vi "uA_build_version.vi"(8 "error in (no error)":errorcluster, 10 "name or relative path":string="Power_Measurement_kit_V2.exe", 11 "path":path) -> (0 "error out":errorcluster, 2 "status":bool, 3 "FileVersion":string)   [LabVIEW 2015]
panel:
  out "string":string
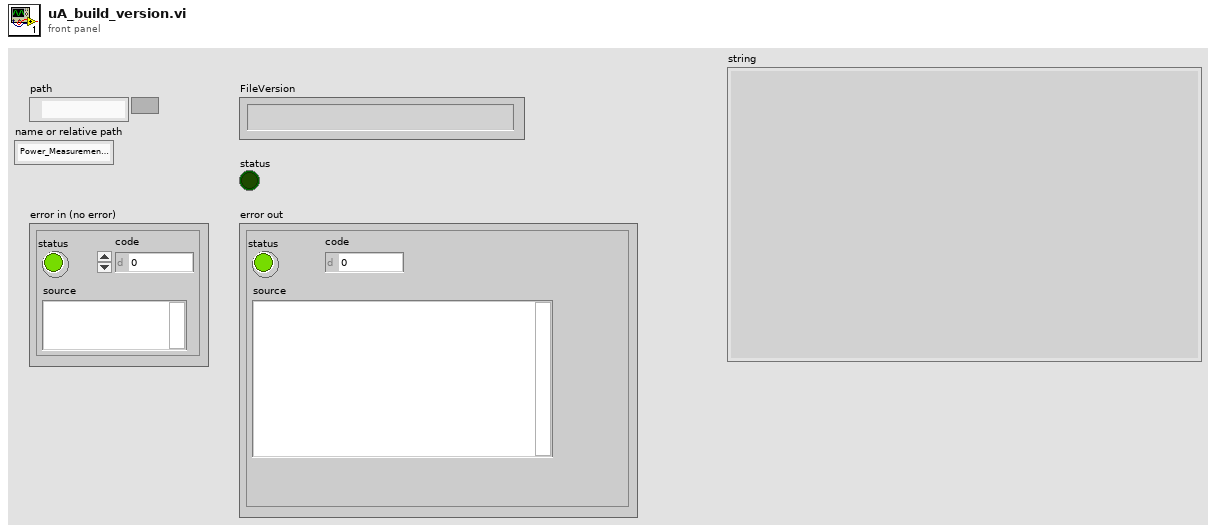
[diagram p1: front panel]
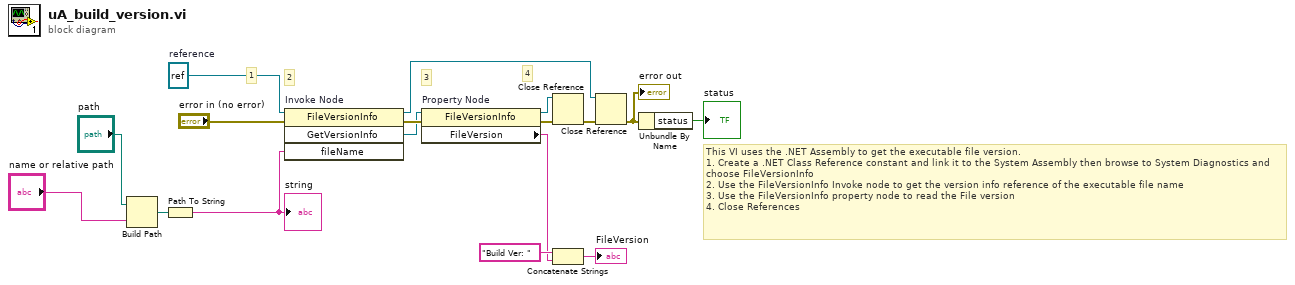
[diagram p0: block diagram]
diagram:
  w4 = refnum<k24> refnum  # reference
  # "4"
  # "3"
  # "2"
  # "1"
  # "This VI uses the .NET Assembly to get the executable file version.\n1. Create a .NET Class Reference constant and link it to the System Assembly then browse to System Diagnostics and choose FileVersionInfo\n2. Use the FileVersionInfo Invoke node to get the version info reference of the executable file name\n3. Use the FileVersionInfo property node to read the File version\n4. Close References"
  n1 = Build Path(base path="path", name or relative path="name or relative path") -> (appended path=w1:path)
  n2 = Path To String(path=w1) -> (string=w5:string)
  "string" <- w5
  n3 = invoke on="Invoke Node" class="FileVersionInfo" method="GetVersionInfo"(reference=w4, error in="error in (no error)", "fileName"=w5) -> (reference out=w11:refnum<k24>, error out=w7:errorcluster, "GetVersionInfo"=w6:refnum<k24>)  [unwired: 1 in, 1 out]
  n4 = property on="Property Node" class="FileVersionInfo"(reference=w6, error in=w7) -> (reference out=w8:refnum<k24>, error out=w9:errorcluster, "FileVersion"=w14:string)
  n5 = Close Reference(reference=w8, error in (no error)=w9) -> (error out=w10:errorcluster)
  n6 = Concatenate Strings("Build Ver: " ("string"), w14) -> (→"FileVersion":string)
  n7 = Close Reference(reference=w11, error in (no error)=w10) -> (error out=w16:errorcluster)
  "error out" <- w16
  n8 = Unbundle By Name(w16) -> ("status"=→"status":bool)
